vi "Add Data.vi"   [LabVIEW 2020, in "SECS Communication.lvlib" / "SECS Data Class.lvclass"]
uses:
  SECS Data Class.lvclass
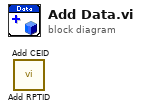
[diagram p0: block diagram]
diagram:
  n1 = call "Add RPTID.vi"() -> ()  [unwired: 11 in, 1 out]
  n2 = call "Add CEID.vi"() -> ()  [unwired: 11 in, 1 out]
